vi "ReadDefaultSubpanel.vi"(6 "timeout in ms (-1)":i32, 8 "error in (no error)":errorcluster, 11 "SMO.UI.MAUI in":refnum<class "SMO.UI.MAUI.lvclass">) -> (0 "error out":errorcluster, 2 "Default Subpanel":refnum<class "SMO.UI.Embedded.lvclass">, 3 "SMO.UI.MAUI out":refnum<class "SMO.UI.MAUI.lvclass">)   [LabVIEW 2019, in "SMO.UI.MAUI.lvclass"]
uses:
  SMO.UI.MAUI.lvclass
  <userlib>/LevyLab/Embedded UI/SMO.UI.Embedded/SMO.UI.Embedded.lvclass
  Typedefs/DefaultSubpanel.ctl
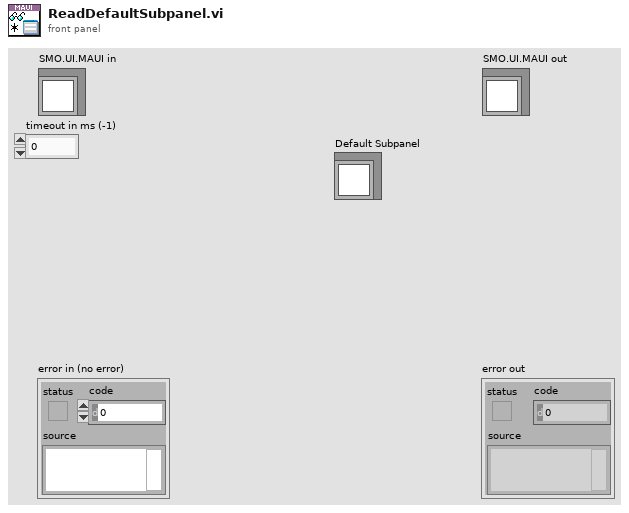
[diagram p1: front panel]
types:
  T1 = typedef "SMO.UI.MAUI.lvclass/DefaultSubpanel.ctl" = cluster{"SMO.UI.Embedded":refnum<class "SMO.UI.Embedded.lvclass">}
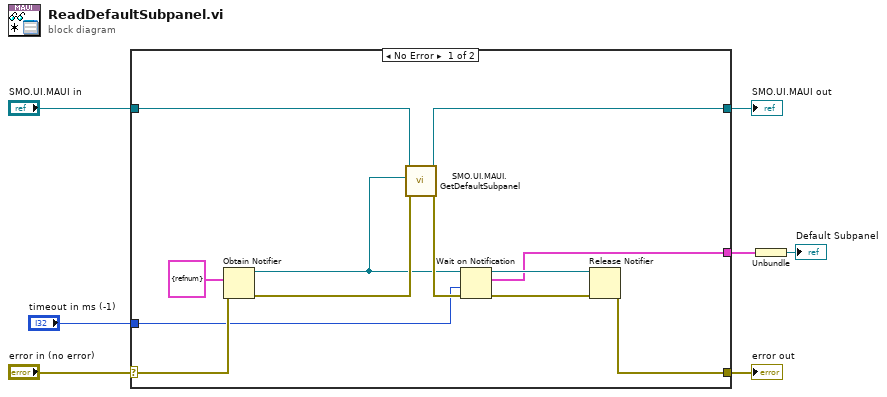
[diagram p0: block diagram]
diagram:
  n1 = case shown="No Error" "error in (no error)" {
    selector: "error in (no error)" -> [w19 w21]
    tunnel: [w15 w21] -> w6
    tunnel: [w8 w20] -> w4
    tunnel: "SMO.UI.MAUI in" -> [w9 w20]
    tunnel: [w11 _] -> w2
    tunnel: "timeout in ms (-1)" -> [w10 _]
    frame No Error {
      n2 = Obtain Notifier(notification data type=T1 {"SMO.UI.Embedded"=refnum} ("Default Subpanel"), error in (no error)=w19) -> (notifier out=w13:refnum<notifier>, error out=w16:errorcluster)  [unwired: 2 in, 1 out]
      n3 = call "SMO.UI.MAUI.GetDefaultSubpanel.vi"("error in (no error)"=w16, "GetDefaultSubpanel"=w13, "SMO.UI.MAUI"=w9) -> ("error out"=w18:errorcluster, "SMO.UI.MAUI out"=w8:refnum<class "SMO.UI.MAUI.lvclass">)  [unwired: 7 in]
      n4 = Wait on Notification(notifier=w13, timeout in ms (-1)=w10, error in (no error)=w18) -> (notifier out=w12:refnum<notifier>, notification=w11:T1, error out=w17:errorcluster)  [unwired: 1 in, 1 out]
      n5 = Release Notifier(notifier=w12, error in (no error)=w17) -> (error out=w15:errorcluster)  [unwired: 1 in, 2 out]
    }
    frame Error {
    }
  }
  "error out" <- w6
  "SMO.UI.MAUI out" <- w4
  n6 = Unbundle(w2) -> ("SMO.UI.Embedded"=→"Default Subpanel":refnum<class "SMO.UI.Embedded.lvclass">)
